vi "Voltmeter.vi"() -> ()   [LabVIEW 2009]
uses:
  <vilib>/DAQmx/create/channels.llb/DAQmx Create Channel (AI-Voltage-Basic).vi
  <vilib>/DAQmx/read.llb/DAQmx Read (Analog DBL 1Chan 1Samp).vi
panel:
  in  "Temperature Sensor Channel":tag
  in  "stop":bool
  out "Meter":dbl(knob) scale=0.0..0.4
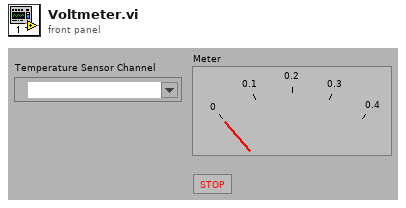
[diagram p1: front panel]
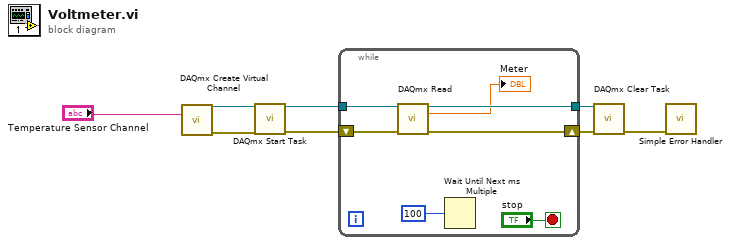
[diagram p0: block diagram]
diagram:
  n1 = call-poly <vilib>:"DAQmx Create Virtual Channel.vi"("physical channels"="Temperature Sensor Channel") -> ("task out"=w3:refnum<k21>, "error out"=w2:errorcluster)  [unwired: 13 in]
  n2 = call <vilib>:"DAQmx Start Task.vi"("task/channels in"=w3, "error in"=w2) -> ("task out"=w8:refnum<k21>, "error out"=w7:errorcluster)  [unwired: 12 in]
  n3 = while {
    tunnel: w8 -> [w14]
    tunnel: [w12] -> w6
    shift-right: [w11] -> w5
    shift-left: w7 -> [w13]
    stop <- "stop" stop-if-true
    n4 = call-poly <vilib>:"DAQmx Read.vi"("task/channels in"=w14, "error in"=w13) -> ("task out"=w12:refnum<k21>, "data"=→"Meter":dbl, "error out"=w11:errorcluster)  [unwired: 11 in]
    n5 = Wait Until Next ms Multiple(millisecond multiple=u32 100 ("Numeric")) -> ()  [unwired: 1 out]
  }
  n6 = call <vilib>:"DAQmx Clear Task.vi"("task in"=w6, "error in"=w5) -> ("error out"=w4:errorcluster)  [unwired: 13 in]
  n7 = call <vilib>:"Simple Error Handler.vi"("error in (no error)"=w4) -> ()  [unwired: 4 in, 5 out]
